vi "test Add-Find-Remove Bus Controller.vi"(8 "error in":errorcluster, 11 "TestCase in":refnum<class "Scripting.lvclass">) -> (0 "error out":errorcluster, 3 "TestCase out":refnum<class "Scripting.lvclass">)   [LabVIEW 2020, in "Scripting.lvclass"]
uses:
  Scripting.lvclass
  C:/dev/git/niveristand-custom-device-testing-tools/VeriStandScriptingTestCase/VeriStandScriptingTestCase.lvclass
  niveristand-custom-device-testing-tools/VeriStandScriptingTestCase/VeriStandScriptingTestCase.lvclass/VeriStandScriptingTestCase.ctl
  niveristand-custom-device-testing-tools/VeriStandScriptingTestCase/Read Target.vi
  NationalInstruments.VeriStand.SystemDefinitionAPI
  <vilib>/addons/_JKI Toolkits/VI Tester/TestCase.llb/TestCase.lvclass
  Scripting/AIM MIL-STD-1553 Scripting.lvlib
  C:/Program Files (x86)/National Instruments/LabVIEW 2020/vi.lib/addons/_JKI Toolkits/VI Tester/TestCase.llb/TestCase.lvclass
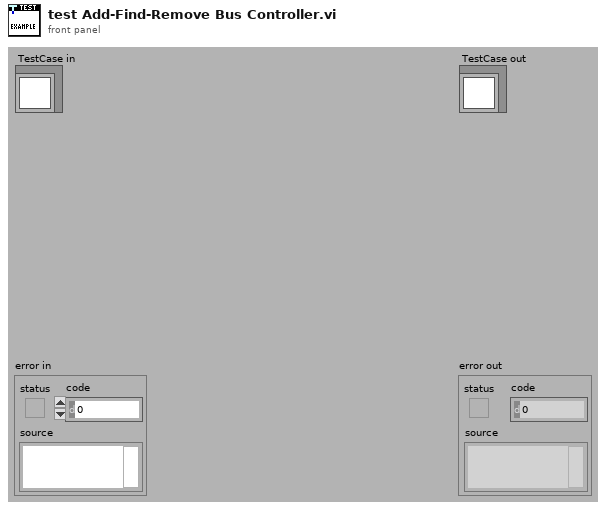
[diagram p1: front panel]
types:
  T1 = typedef "Custom Device API.lvlib/Custom Device Item Ref.ctl" = u64
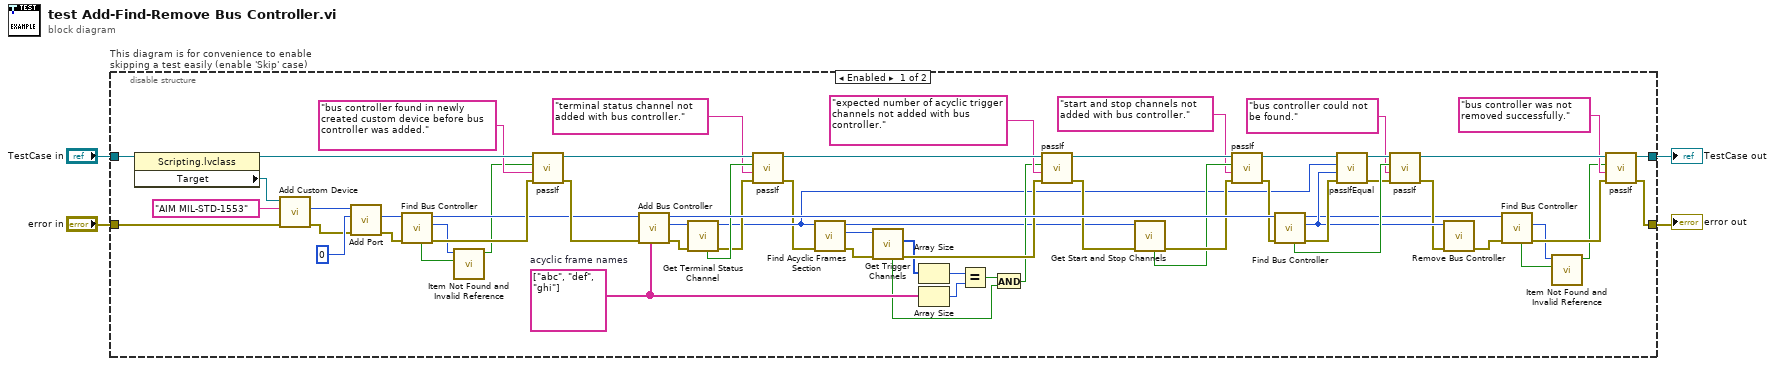
[diagram p0: block diagram]
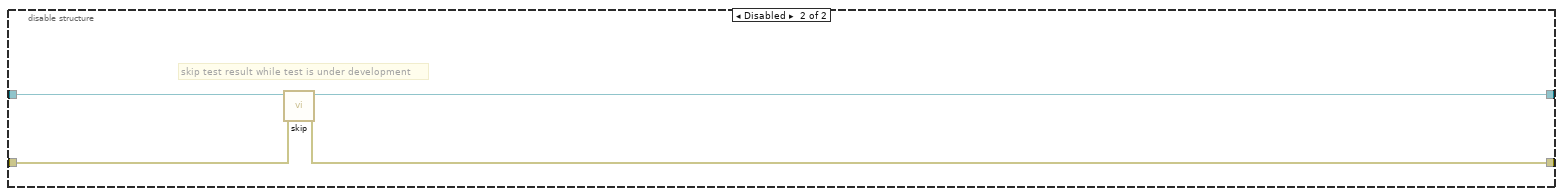
[diagram p2: hidden frame]
diagram:
  n1 = disable-structure "This diagram is for convenience to enable skipping a test easily (enable 'Skip' case)" shown="Enabled" {
    disable-tunnel: "TestCase in" -> [w65 w71]
    disable-tunnel: [w60 w69] -> w1
    disable-tunnel: [w61 w70] -> w3
    disable-tunnel: "error in" -> [w67 w68]
    frame Enabled {
      w32 = string[] ["abc", "def", "ghi"]  # acyclic frame names
      n2 = property class="Scripting.lvclass"(reference=w65) -> (reference out=w44:refnum<class "Scripting.lvclass">, "Target"=w64:refnum<k24>)  [unwired: 1 in, 1 out]
      n3 = call "Add Custom Device.vi"("error in"=w67, "custom device name"="AIM MIL-STD-1553" ("name"), "target"=w64) -> ("error out"=w58:errorcluster, "custom device"=w57:T1)  [unwired: 6 in, 1 out]
      n4 = call "Add Port.vi"("error in"=w58, "port number"=u16 0, "custom device"=w57) -> ("error out"=w55:errorcluster, "port"=w56:T1)  [unwired: 6 in, 1 out]
      n5 = call "Find Bus Controller.vi"("error in"=w55, "port"=w56) -> ("error out"=w53:errorcluster, "bus controller"=w10:T1, "port out"=w43:T1, "found?"=w9:bool)  [unwired: 6 in]
      n6 = call "Item Not Found and Invalid Reference.vi"("found?"=w9, "item reference"=w10) -> ("no item found"=w8:bool)  [unwired: 9 in]
      n7 = call-dynamic "passIf.vi"("error in (no error)"=w53, "message (\"\")"="bus controller found in newly created custom device before bus controller was added.", "pass"=w8, "TestCase in"=w44) -> ("error out"=w54:errorcluster, "TestCase out"=w35:refnum<class "Scripting.lvclass">)  [unwired: 6 in]
      n8 = call "Add Bus Controller.vi"("acyclic frame names"=w32, "error in"=w54, "port"=w43) -> ("error out"=w39:errorcluster, "bus controller"=w38:T1, "port out"=w42:T1)  [unwired: 6 in]
      n9 = call "Get Terminal Status Channel.vi"("error in"=w39, "terminal"=w38) -> ("error out"=w36:errorcluster, "terminal out"=w15:T1, "found?"=w37:bool)  [unwired: 6 in, 1 out]
      n10 = call-dynamic "passIf.vi"("error in (no error)"=w36, "message (\"\")"="terminal status channel not added with bus controller.", "pass"=w37, "TestCase in"=w35) -> ("error out"=w13:errorcluster, "TestCase out"=w34:refnum<class "Scripting.lvclass">)  [unwired: 6 in]
      n11 = call "Find Acyclic Frames Section.vi"("error in"=w13, "bus controller"=w15) -> ("error out"=w12:errorcluster, "acyclic frames section"=w14:T1, "bus controller out"=w11:T1)  [unwired: 6 in, 1 out]
      n12 = call "Get Trigger Channels.vi"("error in"=w12, "acyclic frames section"=w14) -> ("error out"=w41:errorcluster, "acyclic frame triggers"=w40:T1[], "found?"=w21:bool)  [unwired: 6 in, 1 out]
      n13 = Array Size(array=w40) -> (size(s)=w23:i32)
      n14 = Array Size(array=w32) -> (size(s)=w24:i32)
      n15 = Equal?(x=w23, y=w24) -> (x = y?=w22:bool)
      n16 = And(x=w22, y=w21) -> (x .and. y?=w20:bool)
      n17 = call-dynamic "passIf.vi"("error in (no error)"=w41, "message (\"\")"="expected number of acyclic trigger channels not added with bus controller.", "pass"=w20, "TestCase in"=w34) -> ("error out"=w31:errorcluster, "TestCase out"=w30:refnum<class "Scripting.lvclass">)  [unwired: 6 in]
      n18 = call "Get Start and Stop Channels.vi"("error in"=w31, "terminal"=w11) -> ("error out"=w28:errorcluster, "found?"=w26:bool)  [unwired: 5 in, 3 out]
      n19 = call-dynamic "passIf.vi"("error in (no error)"=w28, "message (\"\")"="start and stop channels not added with bus controller.", "pass"=w26, "TestCase in"=w30) -> ("error out"=w16:errorcluster, "TestCase out"=w29:refnum<class "Scripting.lvclass">)  [unwired: 6 in]
      n20 = call "Find Bus Controller.vi"("error in"=w16, "port"=w42) -> ("error out"=w52:errorcluster, "bus controller"=w49:T1, "port out"=w46:T1, "found?"=w51:bool)  [unwired: 6 in]
      n21 = call-dynamic "passIfEqual.vi"("error in (no error)"=w52, "y"=w49, "x"=w15, "TestCase in"=w29) -> ("error out"=w50:errorcluster, "TestCase out"=w62:refnum<class "Scripting.lvclass">)  [unwired: 6 in]
      n22 = call-dynamic "passIf.vi"("error in (no error)"=w50, "message (\"\")"="bus controller could not be found.", "pass"=w51, "TestCase in"=w62) -> ("error out"=w48:errorcluster, "TestCase out"=w59:refnum<class "Scripting.lvclass">)  [unwired: 6 in]
      n23 = call "Remove Bus Controller.vi"("error in"=w48, "bus controller"=w49) -> ("error out"=w47:errorcluster)  [unwired: 9 in]
      n24 = call "Find Bus Controller.vi"("error in"=w47, "port"=w46) -> ("error out"=w45:errorcluster, "bus controller"=w7:T1, "found?"=w6:bool)  [unwired: 6 in, 1 out]
      n25 = call "Item Not Found and Invalid Reference.vi"("found?"=w6, "item reference"=w7) -> ("no item found"=w5:bool)  [unwired: 9 in]
      n26 = call-dynamic "passIf.vi"("error in (no error)"=w45, "message (\"\")"="bus controller was not removed successfully.", "pass"=w5, "TestCase in"=w59) -> ("error out"=w61:errorcluster, "TestCase out"=w60:refnum<class "Scripting.lvclass">)  [unwired: 6 in]
    }
    frame Disabled {
      # "skip test result while test is under development"
      n27 = call <vilib>:"skip.vi"("error in (no error)"=w68, "TestCase in"=w71) -> ("error out"=w70:errorcluster, "TestCase out"=w69:refnum<class "Scripting.lvclass">)  [unwired: 8 in]
    }
  }
  "error out" <- w3
  "TestCase out" <- w1
